vi "All Values.vi"(11 "Entity in":refnum<class "Entity.lvclass">) -> (2 "All Values":refnum<class "Type.lvclass">[](array[class]))   [LabVIEW 2020, in "Conditu2.lvlib" / "Entity.lvclass"]
uses:
  Entity.lvclass
  Columns/Type/Type.lvclass
  Entity.lvclass/Entity.ctl
  Columns/ID/ID.lvclass
  C:/dev/lv20CE/lv-conditum-tools/Conditum-Clone/Columns/Type/Type.lvclass
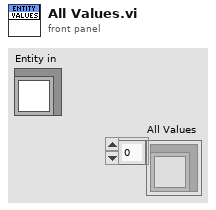
[diagram p1: front panel]
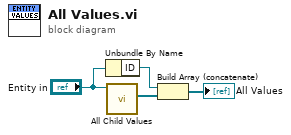
[diagram p0: block diagram]
diagram:
  n1 = Unbundle By Name("Entity in") -> ("ID"=w3:refnum<class "ID.lvclass">)
  n2 = call-dynamic "All Child Values.vi"("Entity in"="Entity in") -> ("All Values"=w2:refnum<class "Type.lvclass">[])  [unwired: 10 in]
  n3 = Build Array (concatenate)(w3, w2) -> (→"All Values":refnum<class "Type.lvclass">[])
